vi "Main.vi"() -> ()   [LabVIEW 2016]
uses:
  <vilib>/Instr/_visa.llb/VISA Configure Serial Port (Serial Instr).vi
panel:
  in  "钳制开关":bool
  in  "开启邮件通知":bool
  out "报警状态":bool
  in  "是否记录工作日志/ .txt":bool
  in  "收件人":string
  in  "开启自动报警":bool
  in  "设置超限阈值":dbl=80.0 format="%#_13g"
  in  "退出":bool
  in  "关闭串口":bool
  in  "打开串口":bool
  out "串口运行状态":bool
  out "平均值":dbl
  out "测量序列":dbl[](array[numeric])
  out "A类不确定度":dbl
  in  "采样频率 f/Hz":string(combo)="5"
  in  "文件存储路径":path=path "C:/Users/dell/Desktop/record_chengming.txt"
  in  "串口配置":T1={"端口"="COM5", "波特率"=9600, "数据位"=8, "奇偶校验"=enum."None"} {"数据位" min=5 max=8 step=1}
  out "实时温度监测":i32(graph)
  # "实时温度监测/T-℃"
  # "设置面板"
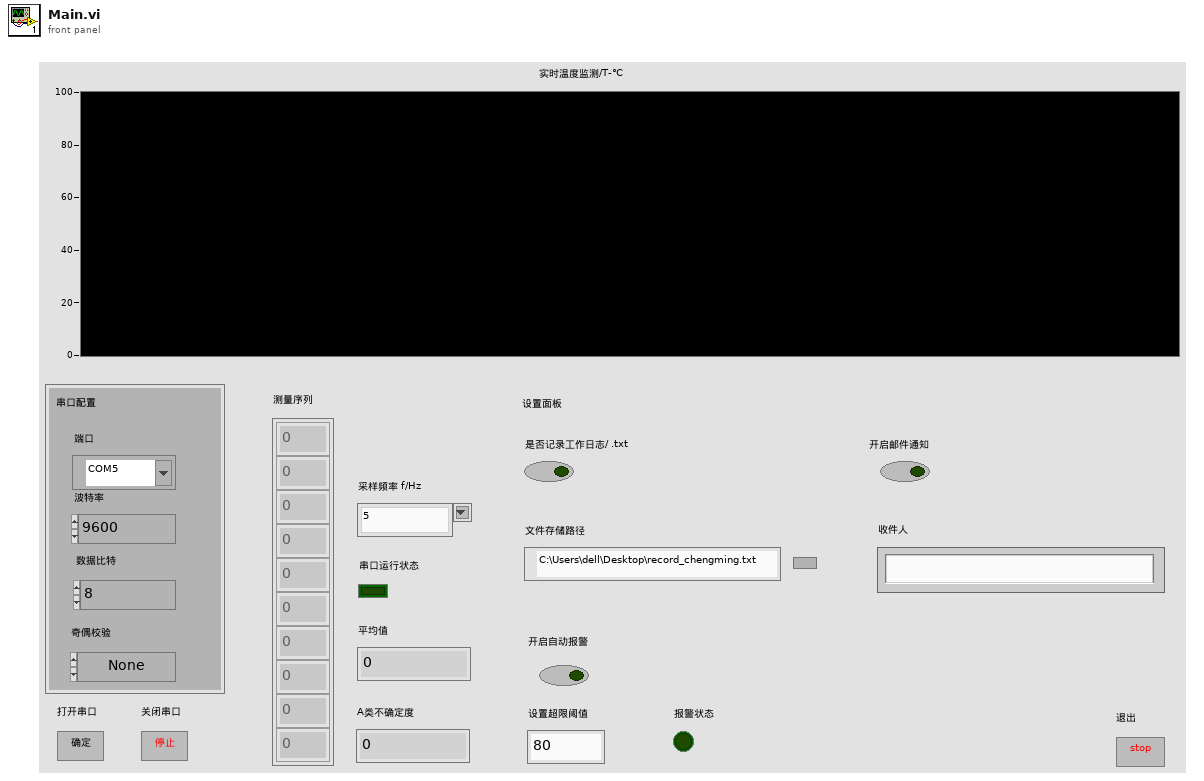
[diagram p1: front panel]
types:
  T1 = cluster{"端口":refnum<visa-resource-name>, "波特率":u32, "数据位":u16, "奇偶校验":enum16{"None", "Odd", "Even", "Mark", "Space"}}
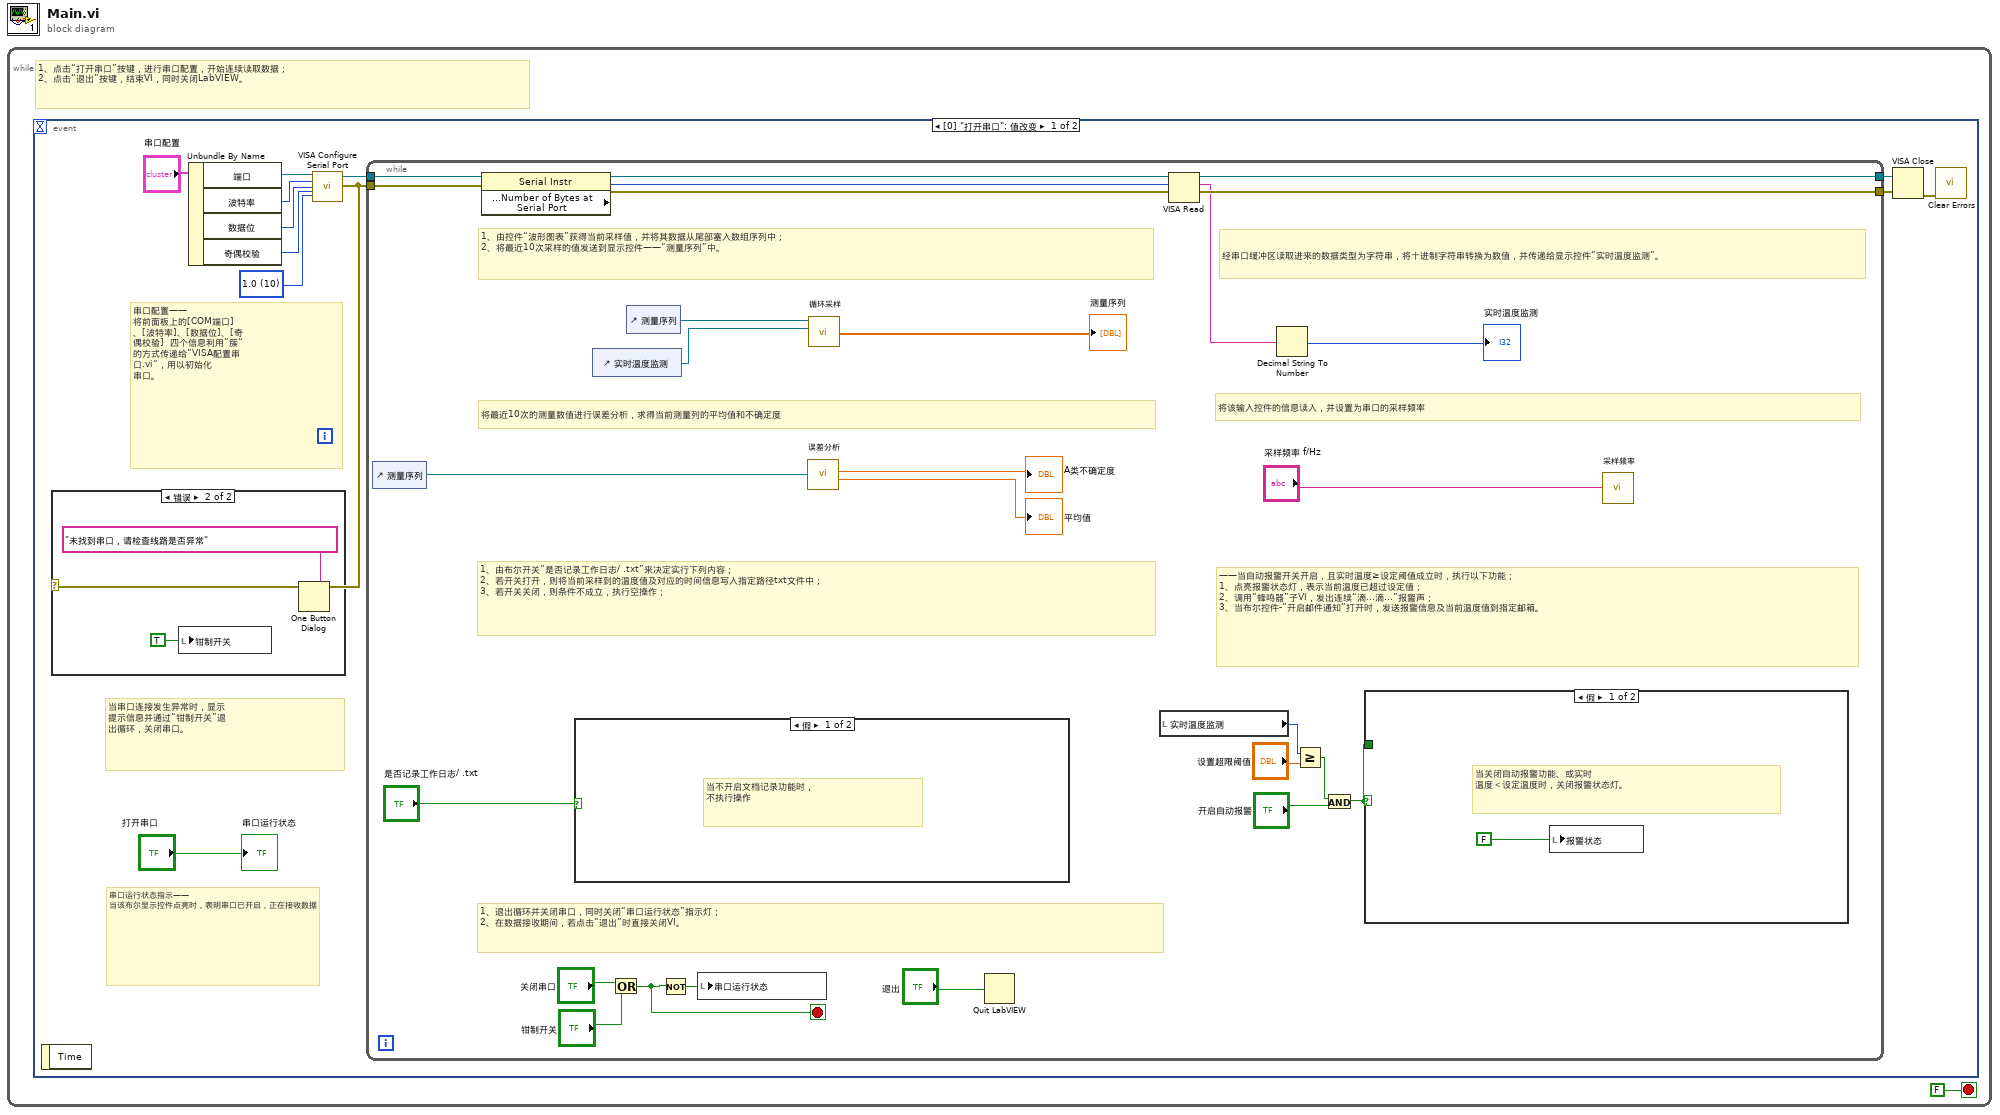
[diagram p0: block diagram]
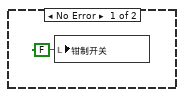
[diagram p2: hidden frame]
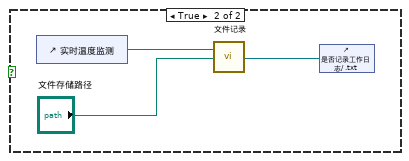
[diagram p3: hidden frame]
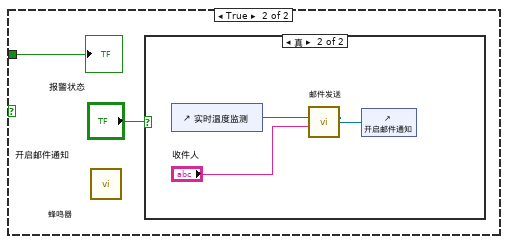
[diagram p4: hidden frame]
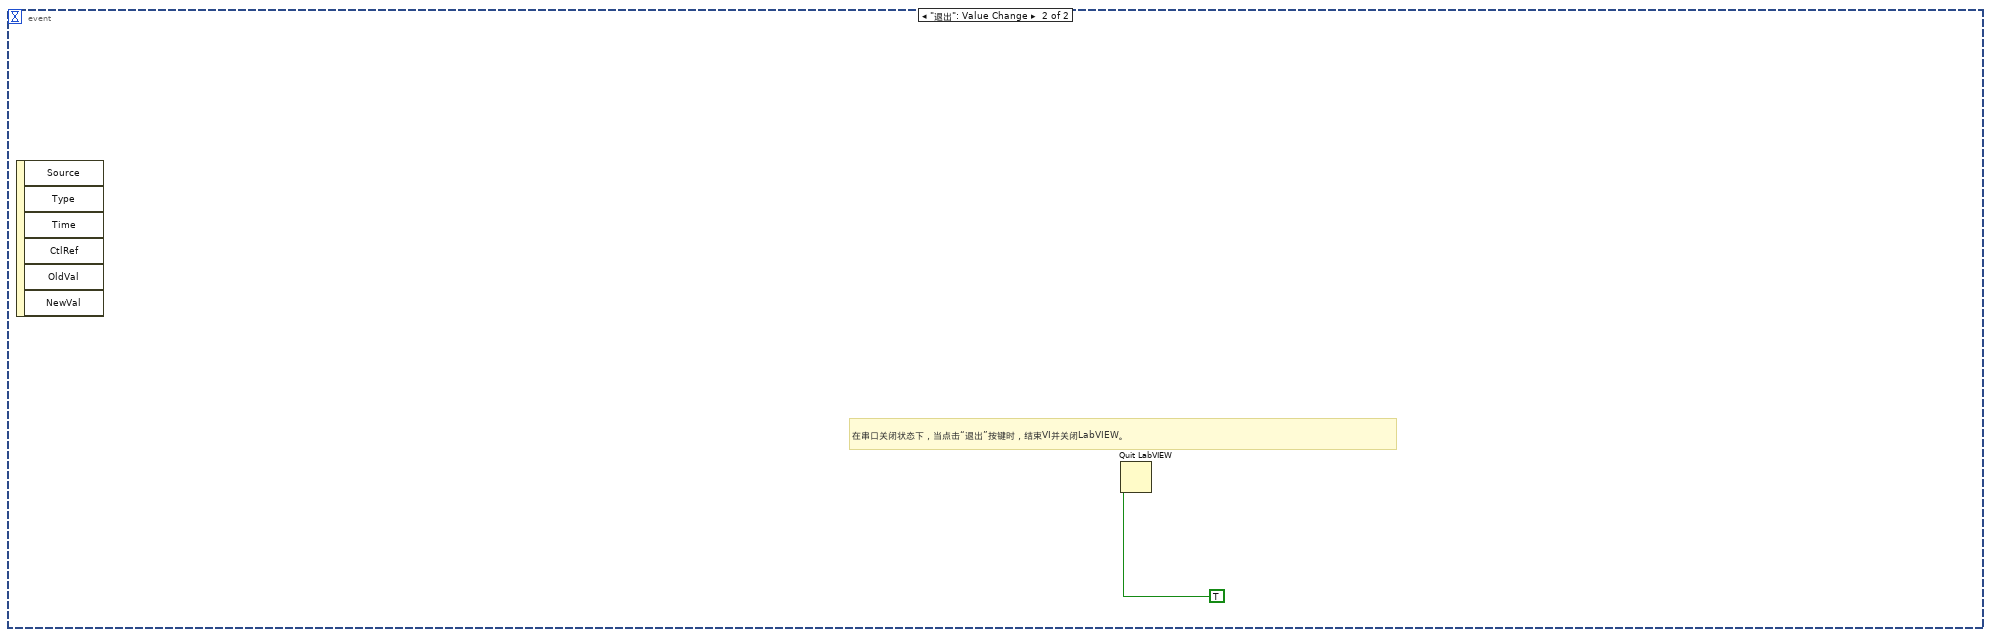
[diagram p6: hidden frame]
diagram:
  n1 = while {
    stop <- FALSE stop-if-true
    # "1、点击“打开串口”按键，进行串口配置，开始连续读取数据；\n2、点击“退出”按键，结束VI，同时关闭LabVIEW。"
    n2 = event "事件结构" shown="[0] \"打开串口\": 值改变" {
      selector: _ -> [_ _]
      dyn-events: _ -> [_ _]
      timeout: _ -> [_ _]
      event "打开串口": Value Change {
        w6 = u16 10 items=["1.0"=10, "1.5"=15, "2.0"=20] ("stop bits (10: 1 bit)")
        # "串口运行状态指示——\n当该布尔显示控件点亮时，表明串口已开启，正在接收数据"
        # "当串口连接发生异常时，显示\n提示信息并通过“钳制开关”退\n出循环，关闭串口。"
        # "串口配置——\n将前面板上的[COM端口]\n、[波特率]、[数据位]、[奇\n偶校验]  四个信息利用“簇“\n的方式传递给”VISA配置串\n口.vi“，用以初始化\n串口。"
        n3 = event-data() -> ()  [unwired: 1 in, 1 out]
        n4 = Unbundle By Name("串口配置") -> ("端口"=w12:refnum<visa-resource-name>, "波特率"=w11:u32, "数据位"=w10:u16, "奇偶校验"=w7:enum16{"None", "Odd", "Even", "Mark", "Space"})
        n5 = call-poly "VISA Configure Serial Port"("VISA resource name"=w12, "baud rate (9600)"=w11, "data bits (8)"=w10, "parity (0:none)"=w7, "stop bits (10: 1 bit)"=w6) -> ("VISA resource name out"=w9:refnum<visa-resource-name>, "error out"=w2:errorcluster)  [unwired: 9 in]
        n6 = case shown="错误" w2 {
          frame No Error {
            n7 = local write "钳制开关"(FALSE) -> ()
          }
          frame Error {
            n8 = local write "钳制开关"(TRUE) -> ()
            n9 = One Button Dialog(message="未找到串口，请检查线路是否异常" ("消息")) -> ()  [unwired: 1 in, 1 out]
          }
        }
        n10 = while {
          tunnel: w9 -> [w29]
          tunnel: w2 -> [w17]
          tunnel: [w28] -> w5
          tunnel: [w27] -> w4
          stop <- w18 stop-if-true
          # "1、退出循环并关闭串口，同时关闭“串口运行状态”指示灯；\n2、在数据接收期间，若点击“退出”时直接关闭VI。"
          # "——当自动报警开关开启，且实时温度≥设定阈值成立时，执行以下功能；\n1、点亮报警状态灯，表示当前温度已超过设定值；\n2、调用“蜂鸣器”子VI，发出连续“滴...滴...”报警声；\n3、当布尔控件-“开启邮件通知”打开时，发送报警信息及当前温度值到指定邮箱。"
          # "将最近10次的测量数值进行误差分析，求得当前测量列的平均值和不确定度"
          # "将该输入控件的信息读入，并设置为串口的采样频率"
          # "1、由布尔开关“是否记录工作日志/ .txt”来决定实行下列内容；\n2、若开关打开，则将当前采样到的温度值及对应的时间信息写入指定路径txt文件中；\n3、若开关关闭，则条件不成立，执行空操作；"
          # "1、由控件“波形图表”获得当前采样值，并将其数据从尾部塞入数组序列中；\n2、将最近10次采样的值发送到显示控件——“测量序列”中。"
          # "经串口缓冲区读取进来的数据类型为字符串，将十进制字符串转换为数值，并传递给显示控件“实时温度监测”。"
          n11 = control-ref of="测量序列"() -> (w24:refnum<vi>)
          n12 = property class="Serial Instr"(reference=w29, error in=w17) -> (reference out=w42:refnum<visa-resource-name>, error out=w41:errorcluster, "Serial Settings:Number of Bytes at Serial Port"=w43:u32)
          n13 = case shown="假" "是否记录工作日志/ .txt" {
            frame False {
              # "当不开启文档记录功能时，\n不执行操作"
            }
            frame True {
              n14 = control-ref of="实时温度监测"() -> (w44:refnum<vi>)
              n15 = control-ref of="是否记录工作日志/ .txt"() -> (w45:refnum<vi>)
              n16 = call "文件记录.vi"("文件存储路径"="文件存储路径", "reference输入"=w44, "Boolean输入"=w45) -> ()  [unwired: 9 in]
            }
          }
          n17 = control-ref of="实时温度监测"() -> (w26:refnum<vi>)
          n18 = Or(x="关闭串口", y="钳制开关") -> (x .or. y?=w18:bool)
          n19 = control-ref of="测量序列"() -> (w30:refnum<vi>)
          n20 = Not(x=w18) -> (.not. x?=w39:bool)
          n21 = local write "串口运行状态"(w39) -> ()
          n22 = call "误差分析.vi"("Array输入"=w24) -> ("平均值"=→"平均值":dbl, "A类不确定度"=→"A类不确定度":dbl)  [unwired: 9 in]
          n23 = call "循环采样.vi"("reference输入"=w26, "Array输入"=w30) -> ("测量序列"=→"测量序列":dbl[])  [unwired: 9 in]
          n24 = Quit LabVIEW(quit? (T)="退出") -> ()
          n25 = local read "实时温度监测"() -> (w23:i32)
          n26 = VISA Read(VISA resource name=w42, byte count=w43, error in (no error)=w41) -> (VISA resource name out=w28:refnum<visa-resource-name>, read buffer=w25:string, error out=w27:errorcluster)  [unwired: 1 out]
          n27 = Decimal String To Number(string=w25) -> (number=→"实时温度监测":i32)  [unwired: 2 in, 1 out]
          n28 = Greater Or Equal?(x=w23, y="设置超限阈值") -> (x >= y?=w37:bool)
          n29 = And(x=w37, y="开启自动报警") -> (x .and. y?=w21:bool)
          n30 = case shown="假" w21 {
            tunnel: w21 -> [_ w48]
            frame False {
              # "当关闭自动报警功能、或实时\n温度＜设定温度时，关闭报警状态灯。"
              n31 = local write "报警状态"(FALSE) -> ()
            }
            frame True {
              n32 = call "蜂鸣器.vi"() -> ()  [unwired: 12 in]
              n33 = case shown="真" "开启邮件通知" {
                frame False {
                  # "当不开启邮件通知功能时，\n不执行操作"
                }
                frame True {
                  n34 = control-ref of="实时温度监测"() -> (w52:refnum<vi>)
                  n35 = control-ref of="开启邮件通知"() -> (w50:refnum<vi>)
                  n36 = call "邮件发送.vi"("收件人"="收件人", "reference输入"=w52, "Boolean输入"=w50) -> ()  [unwired: 9 in]
                }
              }
              "报警状态" <- w48
            }
          }
          n37 = call "采样频率.vi"("采样频率 f/Hz"="采样频率 f/Hz") -> ()  [unwired: 11 in]
        }
        n38 = VISA Close(VISA resource name=w5, error in (no error)=w4) -> (error out=w3:errorcluster)
        n39 = call <vilib>:"Clear Errors.vi"("error in (no error)"=w3) -> ()  [unwired: 5 in, 2 out]
        "串口运行状态" <- "打开串口"
      }
      event "退出": Value Change {
        # "在串口关闭状态下，当点击“退出”按键时，结束VI并关闭LabVIEW。"
        n40 = event-data() -> ()  [unwired: 1 in, 6 out]
        n41 = Quit LabVIEW(quit? (T)=TRUE ("退出？(T)")) -> ()
      }
    }
  }
